vi "Write COM.vi"(8 "error in (no error)":errorcluster, 10 "COM":refnum<visa-resource-name>, 11 "Osciloscopio in":refnum<class "Osciloscopio.lvclass">) -> (0 "error out":errorcluster, 3 "Osciloscopio out":refnum<class "Osciloscopio.lvclass">)   [LabVIEW 2020, in "Oscilloscope.lvlib" / "Osciloscopio.lvclass"]
uses:
  Osciloscopio.lvclass
  Osciloscopio.lvclass/Osciloscopio.ctl
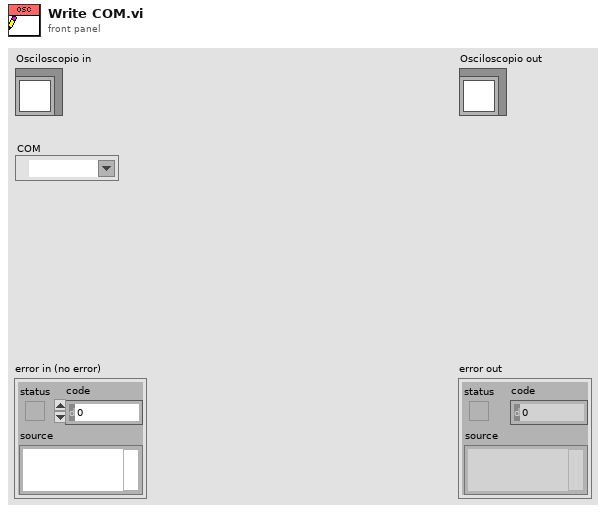
[diagram p1: front panel]
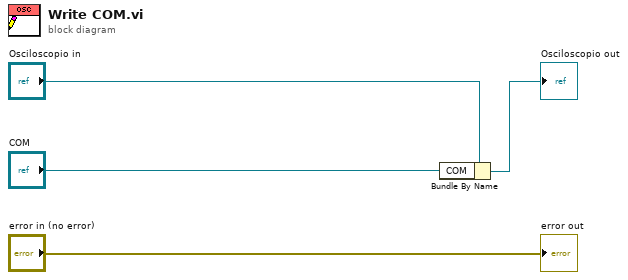
[diagram p0: block diagram]
diagram:
  n1 = Bundle By Name(cluster="Osciloscopio in", "COM"="COM") -> (→"Osciloscopio out":refnum<class "Osciloscopio.lvclass">)
  "error out" <- "error in (no error)"
